vi "Command Displacement Diffs.vi"() -> ()   [LabVIEW 2009]
uses:
  lib/Global Data/Actuator Measurment Actions delete me.ctl
  lib/Data Access Objects/Metadata/LBCB Number.ctl
  lib/Launcher/Launcher Actions.ctl
  lib/Launcher/NoPanelAppTypes.ctl
panel:
  out "Actuator DOF Labels 2":string[](array[string])=["X1", "X2", "Y1", "Z1", "Z2", "Z3"]
  out "AB Diff L2":dbl[](array[numeric]) caption="Differences"
  out "Forces L2":dbl[](array[numeric]) caption="Forces & Moments"
  out "Actuator DOF Labels":string[](array[string])=["X1", "X2", "Y1", "Z1", "Z2", "Z3"]
  in  "Ok":bool
  out "AB Diff L1":dbl[](array[numeric]) caption="Differences"
  out "Forcees L1":dbl[](array[numeric]) caption="Forces & Moments"
  # "LBCB 1"
  # "LBCB 2"
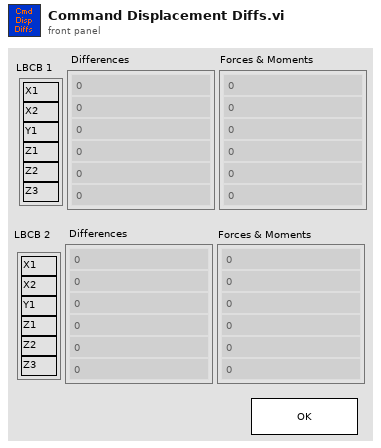
[diagram p1: front panel]
types:
  T1 = typedef "LBCB Number.ctl" = enum16{"LBCB1", "LBCB2"}
  T2 = typedef "Actuator Measurment Actions delete me.ctl" = enum16{"Set  Data", "Get", "Init"}
  T3 = typedef "Actuator DataType.ctl" = cluster{"LVDTs":dbl[], " Commands":dbl[], "Load Cells":dbl[], "Servo":dbl[]}
  T4 = typedef "NoPanelAppTypes.ctl" = enum16{"NTCP Socket", "Data Archiving", "DAQ Link", "Control Loops", "Cmd Disp Diffs", "Individual Readings", "Limits", "Mixed Mode Widget"}
  T5 = typedef "Launcher Actions.ctl" = enum16{"Launch", "Stop All", "Stop", "Kill", "Running?", "Init"}
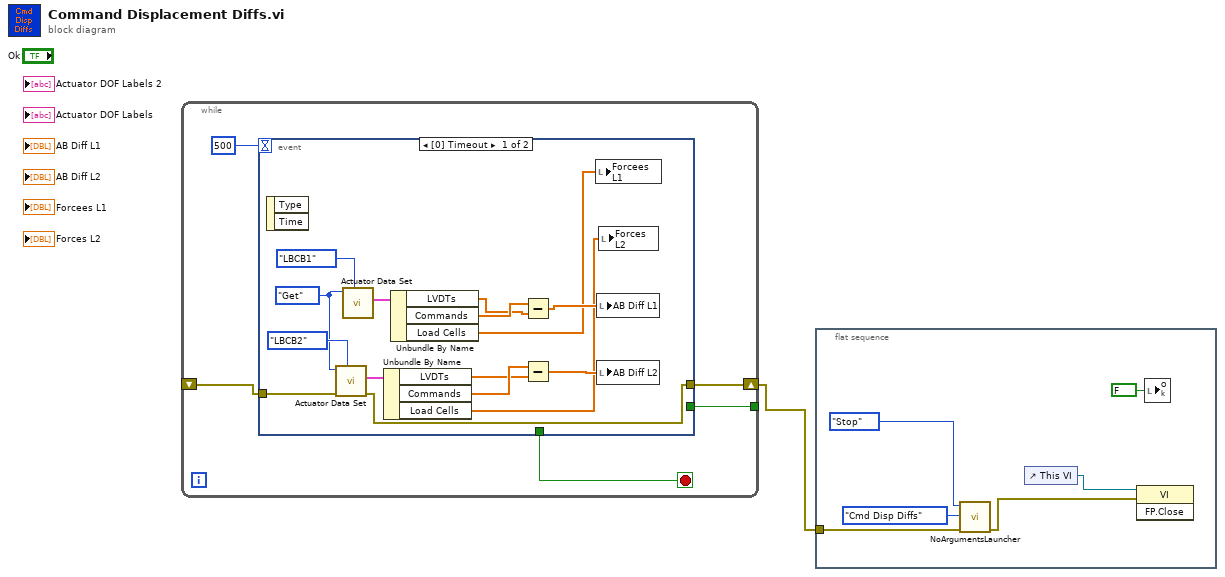
[diagram p0: block diagram]
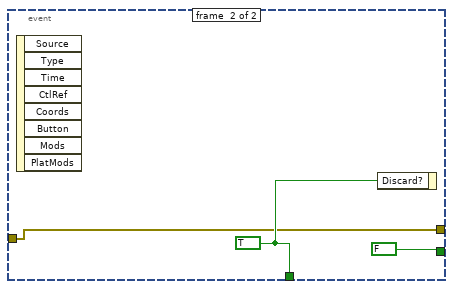
[diagram p2: hidden frame]
diagram:
  n1 = while {
    tunnel: [w4] -> _
    shift-right: [w2] -> w1
    shift-left: _ -> [w3]
    stop <- w5 stop-if-true
    n2 = event shown="[0] Timeout" {
      selector: _ -> [_ _]
      dyn-events: _ -> [_ _]
      timeout: 500 -> [_ _]
      tunnel: [_ w23] -> w5
      tunnel: [_ FALSE] -> w4
      tunnel: w3 -> [w8 w22]
      tunnel: [w7 w22] -> w2
      event #0 {
        w15 = Actuator_Measurment_Actions_delete_me."Get" ("Measurement Actions")
        n3 = event-data() -> ()  [unwired: 3 out]
        n4 = call "Actuator Data Set.vi"("Selected LBCB"=LBCB_Number."LBCB2", "error in (no error)"=w8, "DAO Actions"=w15) -> ("error out"=w7:errorcluster, "Actuator Data Out"=w17:T3)  [unwired: 2 in, 5 out]
        n5 = call "Actuator Data Set.vi"("Selected LBCB"=LBCB_Number."LBCB1", "DAO Actions"=w15) -> ("Actuator Data Out"=w21:T3)  [unwired: 3 in, 6 out]
        n6 = Unbundle By Name(w17) -> ("LVDTs"=w11:dbl[], "Commands"=w14:dbl[], "Load Cells"=w9:dbl[])
        n7 = Unbundle By Name(w21) -> ("LVDTs"=w12:dbl[], "Commands"=w20:dbl[], "Load Cells"=w10:dbl[])
        n8 = Subtract(x=w20, y=w12) -> (x-y=w19:dbl[])
        n9 = Subtract(x=w14, y=w11) -> (x-y=w13:dbl[])
        n10 = local write "Forcees L1"(w10) -> ()
        n11 = local write "AB Diff L1"(w19) -> ()
        n12 = local write "AB Diff L2"(w13) -> ()
        n13 = local write "Forces L2"(w9) -> ()
      }
      event #1 {
        w23 = TRUE
        n14 = event-data() -> ()  [unwired: 9 out]
        n15 = event-data("Discard?"=w23) -> ()  [unwired: 1 in, 1 out]
      }
    }
  }
  n16 = flat-sequence {
    tunnel: w1 -> [w30]
    frame #0 {
      n17 = call "NoArgumentsLauncher.vi"("error in (no error)"=w30, "Application"=NoPanelAppTypes."Cmd Disp Diffs", "Application Launcher Actions"=Launcher_Actions."Stop") -> ("error out"=w26:errorcluster)  [unwired: 8 out]
      n18 = control-ref of="This VI"() -> (w29:refnum<vi>)
      n19 = invoke class="VI" method="FP.Close"(reference=w29, error in=w26) -> ()  [unwired: 1 in, 3 out]
      n20 = local write "Ok"(FALSE ("Ok")) -> ()
    }
  }
